vi "Get DTC Masks.vi"(8 "error in (no error)":errorcluster, 11 "Device Item Ref in":T2 format="%.0x") -> (0 "error out":errorcluster, 2 "DTCs":T1[](array[typedef]), 3 "Device Item Ref out":T2=18446744073709551615 format="%.0x")   [LabVIEW 2013, in "Diagnostics Addon Shared.lvlib"]
uses:
  Diagnostics Addon Shared.lvlib
  <vilib>/NI Veristand/Custom Device API/Custom Device Item Ref.ctl
  DTC Parameters.ctl
  GUID Lookup.vi
  <vilib>/NI Veristand/Custom Device API/Get Item Property (Variant).vi
  <vilib>/NI Veristand/Custom Device API/Custom Device API.lvlib
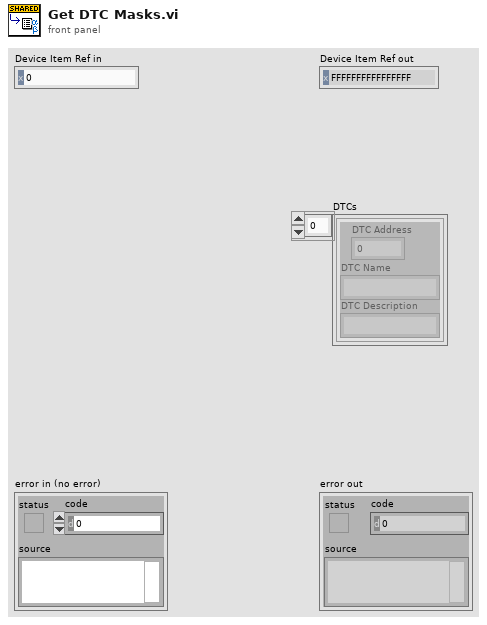
[diagram p1: front panel]
types:
  T1 = typedef "Diagnostics Addon Shared.lvlib/DTC Parameters.ctl" = cluster{"DTC Address":i32, "DTC Name":string, "DTC Description":string}
  T2 = typedef "Custom Device API.lvlib/Custom Device Item Ref.ctl" = u64
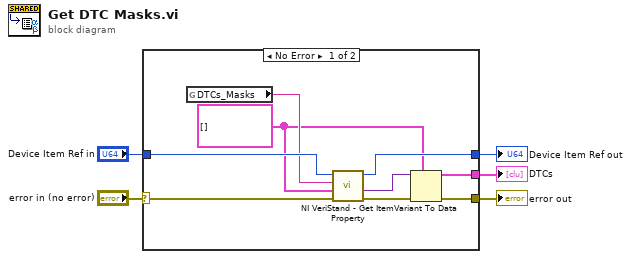
[diagram p0: block diagram]
diagram:
  n1 = case shown="No Error" "error in (no error)" {
    selector: "error in (no error)" -> [w14 w15]
    tunnel: "Device Item Ref in" -> [w13 w16]
    tunnel: [w11 w16] -> w2
    tunnel: [w9 w15] -> w3
    tunnel: [w7 _] -> w1
    frame No Error {
      w6 = T1[] [] ("DTCs")
      n2 = global read "GUID Lookup.vi" "DTCs_Masks"() -> (w12:string)
      n3 = call-poly <vilib>:"NI VeriStand - Get Item Property.vi"("error in (no error)"=w14, "Default Value"=w6, "Property Name"=w12, "Item Ref in"=w13) -> ("error out"=w10:errorcluster, "Value"=w8:variant, "Item Ref out"=w11:T2)  [unwired: 4 in, 1 out]
      n4 = Variant To Data(error in=w10, type=w6, Variant=w8) -> (data=w7:T1[], error out=w9:errorcluster)
    }
    frame Error {
    }
  }
  "error out" <- w3
  "Device Item Ref out" <- w2
  "DTCs" <- w1
